vi "状态监测.vi"(11 "添加的数组":refnum<vi>[](array[refnum])) -> ()   [LabVIEW 2017]
uses:
  <vilib>/Utility/miscctls.llb/LVForegroundBackgroundColorsTypeDef.ctl
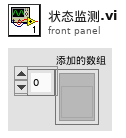
[diagram p1: front panel]
types:
  T1 = typedef "LVForegroundBackgroundColorsTypeDef.ctl" = cluster{"Foreground Color":u32, "Background Color":u32}
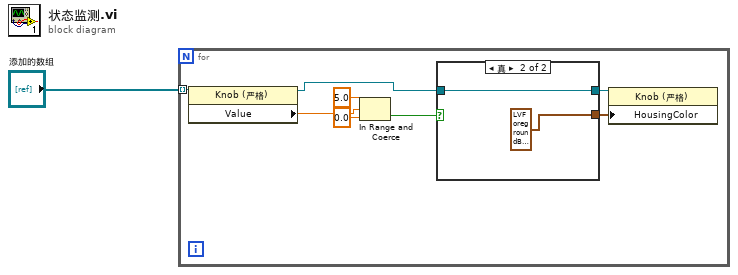
[diagram p0: block diagram]
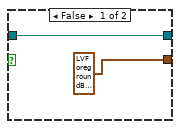
[diagram p2: hidden frame]
diagram:
  n1 = for {
    tunnel: "添加的数组" -> [w9] mode=indexing
    n2 = property class="Knob (严格)"(reference=w9) -> (reference out=w4:refnum<vi>, "Value"=w8:dbl)  [unwired: 1 in, 1 out]
    n3 = In Range and Coerce(upper limit=5.0 ("上限"), x=w8, lower limit=0.0 ("下限")) -> (In Range?=w5:bool)  [unwired: 1 out]
    n4 = case shown="真" w5 {
      tunnel: w4 -> [w10 w13]
      tunnel: [w10 w13] -> w3
      tunnel: [T1 {"Foreground Color"=16711680, "Background Color"=16711680} ("衬底颜色") T1 {"Foreground Color"=6618880, "Background Color"=6618880} ("衬底颜色")] -> w2
      frame False {
      }
      frame True {
      }
    }
    n5 = property class="Knob (严格)"(reference=w3, "HousingColor"=w2) -> ()  [unwired: 1 in, 2 out]
  }
